vi "阶乘构成的数列之和.vi"(11 "n":i32=100) -> (3 "Sn":i32)   [LabVIEW 2012]
doc: "功能：\n\n求1..n之间的所有阶乘之和。\n\n公式：\n\nSn=1!+2!+3!+...n!\n\ncsxcs_366创建"
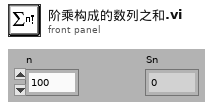
[diagram p1: front panel]
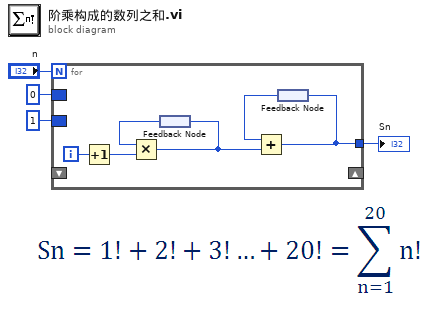
[diagram p0: block diagram]
diagram:
  n1 = for {
    N: "n" -> [_]
    tunnel: [w6] -> w3
    border: 1 -> [_]
    border: 0 -> [_]
    shift-right: _ -> [_]
    shift-left: _ -> [_]
    i -> [w10]
    n2 = Increment(x=w10) -> (x+1=w9:i32)
    n3 = feedback #1() -> (w8:i32)
    n4 = Multiply(x=w8, y=w9) -> (x*y=w5:i32)
    n5 = feedback-in #1(w5) -> ()
    n6 = feedback #2() -> (w7:i32)
    n7 = Add(x=w7, y=w5) -> (x+y=w6:i32)
    n8 = feedback-in #2(w6) -> ()
  }
  "Sn" <- w3
